vi "SetAlarm.vi"(10 "Cluster 2":T1) -> (2 "Cluster":T1)   [LabVIEW 2010]
uses:
  DataCluster.ctl
panel:
  in  "鬧鐘鈴聲":path
  in  "確認":bool
  in  "Time Stamp":timestamp
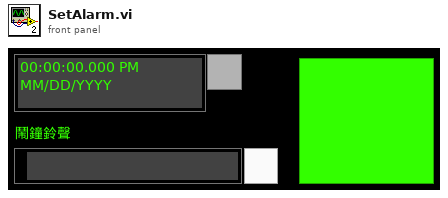
[diagram p1: front panel]
types:
  T1 = typedef "DataCluster.ctl" = cluster{"鬧鐘時間":timestamp, "鈴聲":path, "error ":errorcluster, "Min":dbl, "Sec":dbl, "鬧鐘作用":bool}
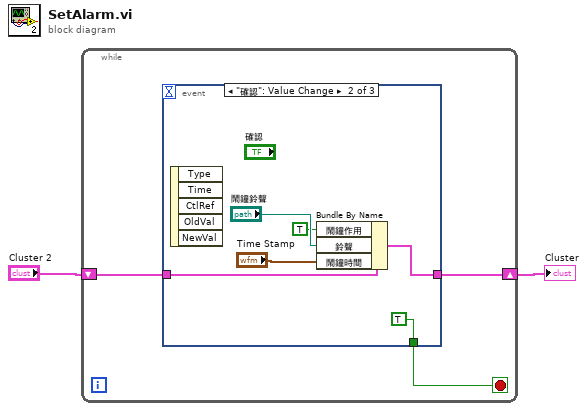
[diagram p0: block diagram]
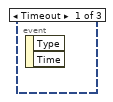
[diagram p2: hidden frame]
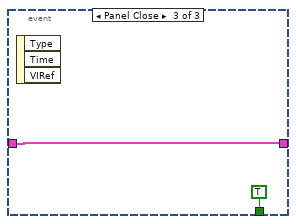
[diagram p3: hidden frame]
diagram:
  n1 = while {
    shift-right: [w4] -> w1
    shift-left: "Cluster 2" -> [w5]
    stop <- w3 stop-if-true
    n2 = event shown="[1] \"確認\": Value Change" {
      selector: _ -> [_ _ _]
      dyn-events: _ -> [_ _ _]
      timeout: _ -> [_ _ _]
      tunnel: w5 -> [_ w11 w13]
      tunnel: [_ w8 w13] -> w4
      tunnel: [_ TRUE TRUE] -> w3
      event Timeout {
        n3 = event-data() -> ()  [unwired: 1 in, 2 out]
      }
      event "確認": Value Change {
        n4 = event-data() -> ()  [unwired: 1 in, 5 out]
        n5 = Bundle By Name(cluster=w11, "鬧鐘作用"=TRUE, "鈴聲"="鬧鐘鈴聲", "鬧鐘時間"="Time Stamp") -> (w8:T1)
      }
      event Panel Close {
        n6 = event-data() -> ()  [unwired: 1 in, 3 out]
      }
    }
  }
  "Cluster" <- w1
